vi "1Cx2x3-Small RC.vi"() -> ()   [LabVIEW 2011]
uses:
  2-RIO/2 Typedefs/Which Boat.ctl
  Classes/TCP Connections/TCP Small Boat/TCP Small Boat.lvclass
  2-RIO/2 Typedefs/sensorData.ctl
  2-RIO/2 Typedefs/UTM Location.ctl
  2-RIO/2 Typedefs/heading.ctl
  2-RIO/2 Globals/2 Global.vi
  Classes/Missions/MissionQueue/MissionQueue.lvclass
panel:
  in  "remote port or service name":u16=10001
  in  "address":string="192.168.1.11"
  out "E-stop freq.":dbl
  out "Act freq.":dbl
  out "Sense freq.":dbl
  out "OCU freq.":dbl
  out "RIO freq.":dbl
  in  "E-Stop":bool
  in  "Sense Data Source":enum16{"Overhead Camera", "Simulation"}(ring)
  # "this is the parent VI under which \nthe Small RC Boat's sensors, RIO and OCU run."
  # "TODO: check to see that these frequencies are actually\nbeing measured right"
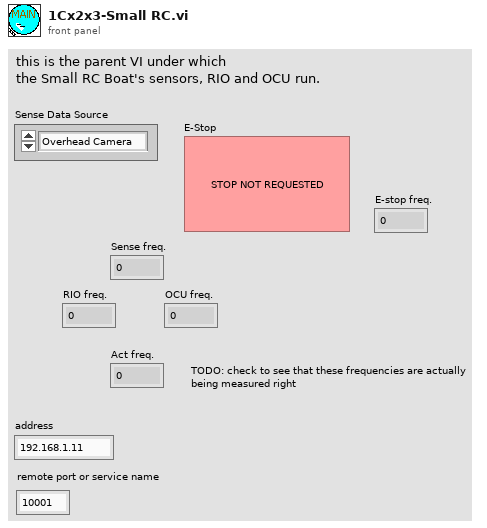
[diagram p1: front panel]
types:
  T1 = typedef "sensorData.ctl" = cluster{"Boat Location":T2, "Robot Heading ":T3, "Wind Speed":dbl, "Wind Direction":T3}
  T2 = typedef "UTM Location.ctl" = cluster{"UTM Zone":dbl, "Hemisphere":enum16{"North", "South"}, "East":dbl, "North":dbl}
  T3 = typedef "heading.ctl" = dbl
  T4 = typedef "Which Boat.ctl" = u16
  T5 = typedef "apparent wind direction.ctl" = dbl
  T6 = typedef "apparent wind speed.ctl" = dbl
  T7 = typedef "manual override.ctl" = cluster{"Override Active":bool, "Setpoints":T8}
  T8 = typedef "setpoints to boat.ctl" = cluster{"Sail Position":T9, "Rudder Angle":T10}
  T9 = typedef "sail setpt.ctl" = dbl
  T10 = typedef "rudder angle.ctl" = dbl
  T11 = typedef "IMAQ Image.ctl" = refnum<image>
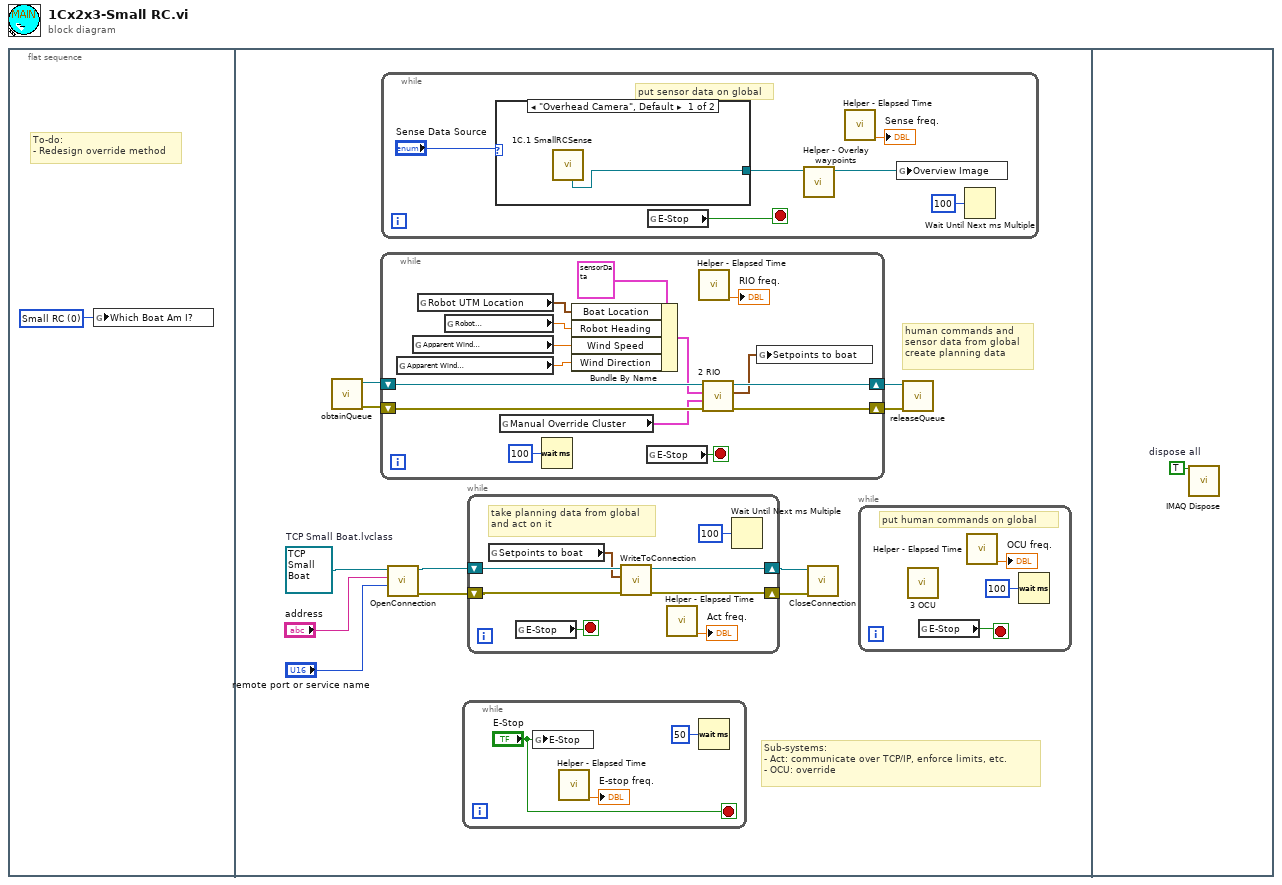
[diagram p0: block diagram]
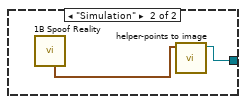
[diagram p2: hidden frame]
diagram:
  n1 = flat-sequence {
    frame #0 {
      w1 = T4 0 items=["Small RC", "Large RC", "Final Boat", "Simulator"] ("Which Boat Am I?")
      # "To-do:\n- Redesign override method"
      n2 = global write "2 Global.vi" "Which Boat Am I?"(w1) -> ()
    }
    frame #1 {
      w12 = refnum<class "TCP Small Boat.lvclass"> refnum  # TCP Small Boat.lvclass
      # "human commands and \nsensor data from global\ncreate planning data"
      # "Sub-systems:\n- Act: communicate over TCP/IP, enforce limits, etc.\n- OCU: override"
      n3 = call "obtainQueue.vi"() -> ("Error Out"=w5:errorcluster, "MissionQueue.lvclass"=w4:refnum<class "MissionQueue.lvclass">)  [unwired: 10 in]
      n4 = while {
        shift-right: [w28] -> w3
        shift-left: w4 -> [w30]
        shift-right: [w27] -> w2
        shift-left: w5 -> [w26]
        stop <- w32 stop-if-true
        n5 = global read "2 Global.vi" "Apparent Wind\nDirection"() -> (w21:T5)
        n6 = global read "2 Global.vi" "Apparent Wind\nSpeed"() -> (w22:T6)
        n7 = global read "2 Global.vi" "Robot UTM Location"() -> (w23:T2)
        n8 = global read "2 Global.vi" "Robot\nHeading"() -> (w20:T3)
        n9 = global read "2 Global.vi" "Manual Override Cluster"() -> (w25:T7)
        n10 = Wait (ms)(milliseconds to wait=u32 100 ("millisecond multiple")) -> ()  [unwired: 1 out]
        n11 = Bundle By Name(cluster=T1 {"Boat Location"={"UTM Zone"=0.0, "Hemisphere"=enum."North", "East"=0.0, "North"=0.0}, "Robot Heading "=0.0, "Wind Speed"=0.0, "Wind Direction"=0.0} ("Sensor Data"), "Boat Location"=w23, "Robot Heading"=w20, "Wind Speed"=w22, "Wind Direction"=w21) -> (w24:T1)
        n12 = global read "2 Global.vi" "E-Stop"() -> (w32:bool)
        n13 = call "Helper - Elapsed Time.vi"() -> ("Frequency (Hz)"=→"RIO freq.":dbl)  [unwired: 10 in, 1 out]
        n14 = call "2 RIO.vi"("Error In"=w26, "Manual Override Cluster"=w25, "Sensor Data"=w24, "MissionQueue In"=w30) -> ("Error Out"=w27:errorcluster, "Setpoints to Boat"=w19:T8, "MissionQueue Out"=w28:refnum<class "MissionQueue.lvclass">)  [unwired: 5 in]
        n15 = global write "2 Global.vi" "Setpoints to boat"(w19) -> ()
      }
      n16 = while {
        stop <- w46 stop-if-true
        # "put sensor data on global"
        n17 = case shown="\"Overhead Camera\", Default" "Sense Data Source" {
          tunnel: [w48 w49] -> w43
          frame "Overhead Camera", Default {
            n18 = call "1C.1 SmallRCSense.vi"() -> ("Eye in the Sky"=w48:T11)  [unwired: 6 in, 5 out]
          }
          frame "Simulation" {
            n19 = call "1B Spoof Reality.vi"() -> ("Boat Path"=w50:cluster{"X Position":dbl, "Y Position":dbl}[])  [unwired: 5 in, 6 out]
            n20 = call "helper-points to image.vi"("Array of Points"=w50) -> ("Image Out"=w49:T11)  [unwired: 10 in]
          }
        }
        n21 = global read "2 Global.vi" "E-Stop"() -> (w46:bool)
        n22 = call "Helper - Overlay waypoints.vi"("Img Refnum in"=w43) -> ("Img Refnum out"=w44:T11)  [unwired: 10 in]
        n23 = call "Helper - Elapsed Time.vi"() -> ("Frequency (Hz)"=→"Sense freq.":dbl)  [unwired: 10 in, 1 out]
        n24 = global write "2 Global.vi" "Overview Image"(w44) -> ()
        n25 = Wait Until Next ms Multiple(millisecond multiple=u32 100) -> ()  [unwired: 1 out]
      }
      n26 = call-dynamic "OpenConnection.vi"("remote port or service name"="remote port or service name", "address"="address", "TCP Connection in"=w12) -> ("error out"=w9:errorcluster, "TCP Connection out"=w8:refnum<class "TCP Small Boat.lvclass">)  [unwired: 7 in]
      n27 = while {
        stop <- "E-Stop" stop-if-true
        n28 = global write "2 Global.vi" "E-Stop"("E-Stop") -> ()
        n29 = call "Helper - Elapsed Time.vi"() -> ("Frequency (Hz)"=→"E-stop freq.":dbl)  [unwired: 10 in, 1 out]
        n30 = Wait (ms)(milliseconds to wait=u32 50 ("millisecond multiple")) -> ()  [unwired: 1 out]
      }
      n31 = while {
        shift-right: [w37] -> w6
        shift-left: w9 -> [w38]
        shift-right: [w35] -> w7
        shift-left: w8 -> [w36]
        stop <- w40 stop-if-true
        # "take planning data from global\nand act on it"
        n32 = global read "2 Global.vi" "Setpoints to boat"() -> (w34:T8)
        n33 = global read "2 Global.vi" "E-Stop"() -> (w40:bool)
        n34 = call "WriteToConnection.vi"("error in (no error)"=w38, "Setpoints to boat"=w34, "TCP Small Boat in"=w36) -> ("error out"=w37:errorcluster, "TCP Small Boat out"=w35:refnum<class "TCP Small Boat.lvclass">)  [unwired: 7 in]
        n35 = call "Helper - Elapsed Time.vi"() -> ("Frequency (Hz)"=→"Act freq.":dbl)  [unwired: 10 in, 1 out]
        n36 = Wait Until Next ms Multiple(millisecond multiple=u32 100) -> ()  [unwired: 1 out]
      }
      n37 = call-dynamic "CloseConnection.vi"("error in (no error)"=w6, "TCP Connection in"=w7) -> ()  [unwired: 8 in, 2 out]
      n38 = while {
        stop <- w17 stop-if-true
        # "put human commands on global"
        n39 = call "3 OCU.vi"() -> ()  [unwired: 12 in]
        n40 = global read "2 Global.vi" "E-Stop"() -> (w17:bool)
        n41 = call "Helper - Elapsed Time.vi"() -> ("Frequency (Hz)"=→"OCU freq.":dbl)  [unwired: 10 in, 1 out]
        n42 = Wait (ms)(milliseconds to wait=u32 100 ("millisecond multiple")) -> ()  [unwired: 1 out]
      }
      n43 = call "releaseQueue.vi"("Error In"=w2, "MissionQueue.lvclass"=w3) -> ()  [unwired: 8 in, 2 out]
    }
    frame #2 {
      w51 = TRUE  # dispose all
      n44 = call "IMAQ Dispose"("All Images? (No)"=w51) -> ()  [unwired: 5 in, 1 out]
    }
  }
